vi "img_make_cam.vi"() -> ()   [LabVIEW 2016]
uses:
  <vilib>/userdefined/High Color/IMAQdx.ctl
  <vilib>/vision/driver/NI_Vision_Acquisition_Software.lvlib
  <vilib>/vision/NI_Vision_Development_Module.lvlib
panel:
  out "error out":errorcluster
  in  "save":bool
  in  "X Resolution 2":i32
  in  "Y Resolution 2":i32
  in  "Optional Rectangle":i32[](array[numeric])
  in  "Y Resolution":i32
  in  "X Resolution":i32
  out "Image":T1(plugin-control)
  in  "정지":bool
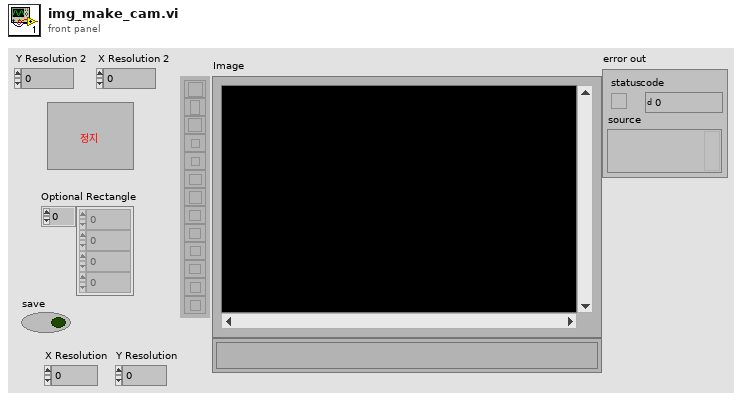
[diagram p1: front panel]
types:
  T1 = typedef "IMAQ Image.ctl" = refnum<image>
  T2 = typedef "IMAQdx.ctl" = refnum<k21>
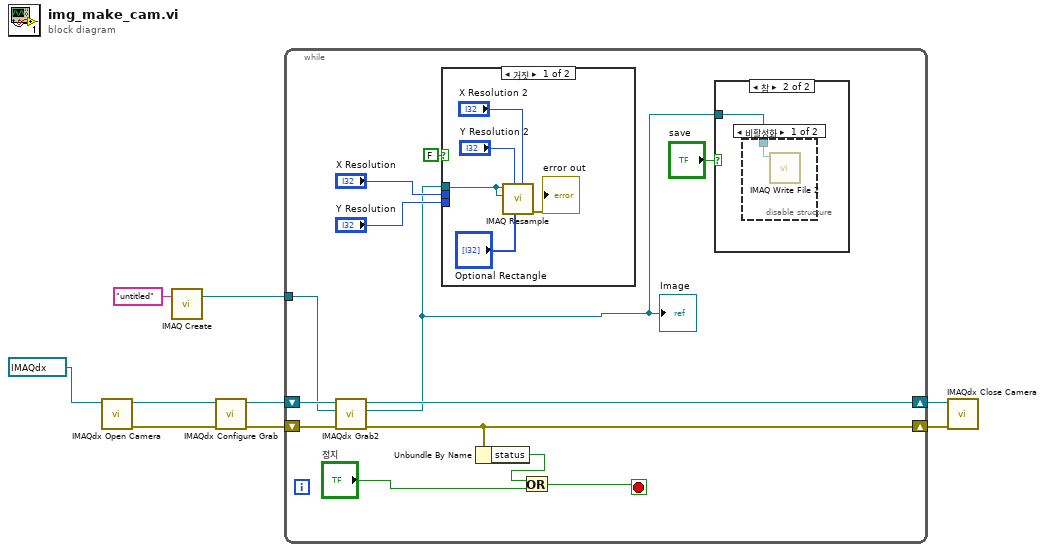
[diagram p0: block diagram]
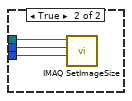
[diagram p4: hidden frame]
diagram:
  n1 = call <vilib>:"IMAQdx Open Camera.vi"("Session In"=T2 "cam0") -> ("error out"=w6:errorcluster, "Session Out"=w9:T2)  [unwired: 9 in]
  n2 = call "IMAQ Create"("Image Name"="untitled") -> ("New Image"=w2:T1)  [unwired: 4 in, 1 out]
  n3 = call <vilib>:"IMAQdx Configure Grab.vi"("error in"=w6, "Session In"=w9) -> ("error out"=w5:errorcluster, "Session Out"=w8:T2)  [unwired: 8 in]
  n4 = while {
    shift-right: [w21] -> w7
    shift-left: w8 -> [w22]
    shift-right: [w19] -> w4
    shift-left: w5 -> [w20]
    tunnel: w2 -> [w15]
    stop <- w18 stop-if-true
    n5 = call <vilib>:"IMAQdx Grab2.vi"("error in"=w20, "Image In"=w15, "Session In"=w22) -> ("error out"=w19:errorcluster, "Image Out"=w10:T1, "Session Out"=w21:T2)  [unwired: 5 in, 1 out]
    "Image" <- w10
    n6 = case shown="거짓" FALSE {
      tunnel: "X Resolution" -> [_ w32]
      tunnel: "Y Resolution" -> [_ w31]
      tunnel: w10 -> [w29 w30]
      frame False {
        n7 = call "IMAQ Resample"("X Resolution"="X Resolution 2", "Optional Rectangle"="Optional Rectangle", "Y Resolution"="Y Resolution 2", "Image Dst"=w29, "Image Src"=w29) -> ("error out"=→"error out":errorcluster)  [unwired: 5 in, 1 out]
      }
      frame True {
        n8 = call "IMAQ SetImageSize"("Y Resolution"=w31, "X Resolution"=w32, "Image"=w30) -> ()  [unwired: 2 in, 2 out]
      }
    }
    n9 = Unbundle By Name(w19) -> ("status"=w17:bool)
    n10 = Or(x=w17, y="정지") -> (x .or. y?=w18:bool)
    n11 = case shown="참" "save" {
      tunnel: w10 -> [_ w23]
      frame False {
      }
      frame True {
        n12 = disable-structure shown="비활성화" {
          disable-tunnel: w23 -> [w24 _]
          frame Disabled {
            n13 = call-poly "IMAQ Write File 2"("Image"=w24) -> ()  [unwired: 9 in, 2 out]
          }
          frame Enabled {
          }
        }
      }
    }
  }
  n14 = call <vilib>:"IMAQdx Close Camera.vi"("error in"=w4, "Session In"=w7) -> ()  [unwired: 9 in, 1 out]
